vi "DG635 Set Channel Delay.vi"(6 "Relative to channel":T1, 7 "Output channel":T1, 8 "error in":errorcluster, 10 "Start delay":dbl format="%#_6ps", 11 "VISA resource name":refnum<visa-resource-name>) -> (0 "error out":errorcluster, 2 "Status byte":i32 format="%b", 3 "VISA resource name out":refnum<visa-resource-name>)   [LabVIEW 2021]
uses:
  DG635 Channel.ctl
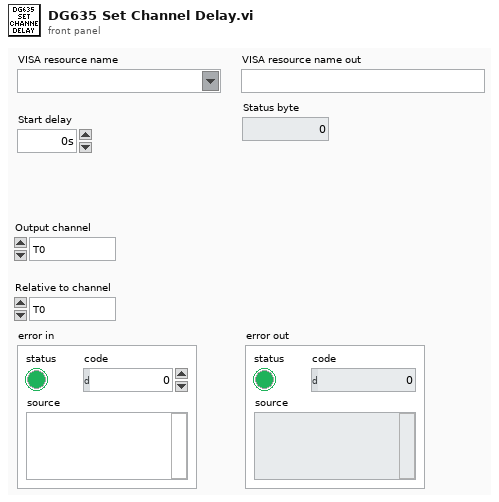
[diagram p1: front panel]
types:
  T1 = typedef "DG635 Channel.ctl" = enum16{"T0", "T1", "A", "B", "C", "D", "E", "F", "G", "H"}
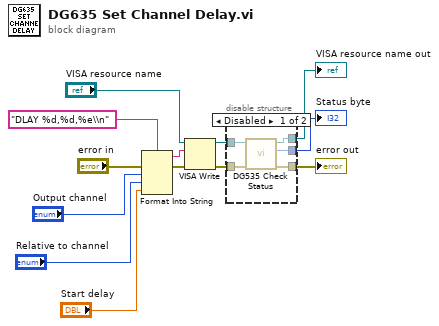
[diagram p0: block diagram]
diagram:
  n1 = Format Into String(format string="DLAY %d,%d,%e\\n", error in="error in", "Output channel", "Relative to channel", "Start delay") -> (resulting string=w6:string, error out=w7:errorcluster)  [unwired: 1 in]
  n2 = VISA Write(VISA resource name="VISA resource name", write buffer=w6, error in (no error)=w7) -> (VISA resource name out=w3:refnum<visa-resource-name>, error out=w5:errorcluster)  [unwired: 1 out]
  n3 = disable-structure shown="Disabled" {
    disable-tunnel: w5 -> [w18 w19]
    disable-tunnel: [w17 w19] -> w4
    disable-tunnel: w3 -> [w16 w20]
    disable-tunnel: [w15 w20] -> w2
    disable-tunnel: [w14 _] -> w1
    frame Disabled {
      n4 = call "DG535 Check Status.vi"("error in"=w18, "VISA resource name"=w16) -> ("error out"=w17:errorcluster, "Status byte"=w14:i32, "VISA resource name out"=w15:refnum<visa-resource-name>)  [unwired: 6 in, 1 out]
    }
    frame Enabled {
    }
  }
  "error out" <- w4
  "VISA resource name out" <- w2
  "Status byte" <- w1
